vi "Init Msg Default.vi"() -> (2 "Msg":refnum<class "Msg.lvclass">)   [LabVIEW 2020, in "_Template.lvlib" / "Templates.lvlib" / "TEMPLATE jettl Msg.lvlib" / "TEMPLATE.lvlib"]
uses:
  TEMPLATE.lvlib
  jettl/jettl/Msg/Msg.lvclass
  TEMPLATE Msg/TEMPLATE Msg.lvlib
panel:
  # "This front panel should not be manipulated."
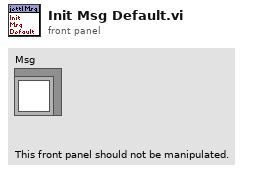
[diagram p1: front panel]
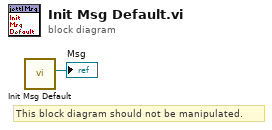
[diagram p0: block diagram]
diagram:
  # "This block diagram should not be manipulated."
  n1 = call "Init Msg Default.vi"() -> ("Msg"=→"Msg":refnum<class "Msg.lvclass">)  [unwired: 11 in]
